vi "Untitled 2.vi"() -> ()   [LabVIEW 2009]
panel:
  in  "VISA resource name":refnum<visa-resource-name>
  out "read buffer":string
  out "return count":u32
  out "error out 2":errorcluster
  out "error out":errorcluster
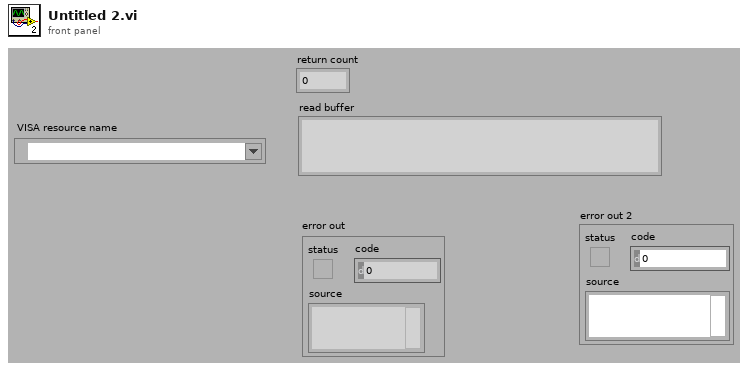
[diagram p1: front panel]
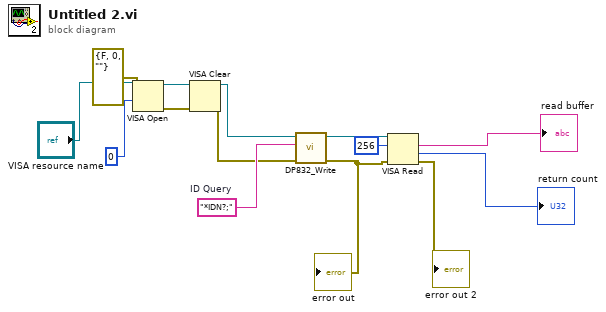
[diagram p0: block diagram]
diagram:
  w14 = "*IDN?;"  # ID Query
  n1 = VISA Open(access mode=u32 0, error in (no error)=errorcluster {"status"=FALSE, "code"=0, "source"=""}, VISA resource name="VISA resource name") -> (VISA resource name=w6:refnum<visa-resource-name>, error out=w5:errorcluster)  [unwired: 2 out]
  n2 = VISA Clear(VISA resource name=w6, error in (no error)=w5) -> (VISA resource name out=w3:refnum<visa-resource-name>, error out=w2:errorcluster)
  n3 = call "DP832_Write.vi"("error in (no error)"=w2, "Write Buffer (\"\")"=w14, "VISA resource name"=w3) -> ("error out"=w12:errorcluster, "VISA resource name out"=w13:refnum<visa-resource-name>)  [unwired: 7 in]
  "error out" <- w12
  n4 = VISA Read(VISA resource name=w13, byte count=u32 256, error in (no error)=w12) -> (read buffer=→"read buffer":string, return count=→"return count":u32, error out=→"error out 2":errorcluster)  [unwired: 1 out]
